vi "Get Default Configuration.vi"() -> (2 "Configuration":T1)   [LabVIEW 2014, in "System.lvclass"]
uses:
  System.lvclass
  Configuration - cluster.ctl
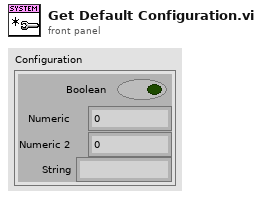
[diagram p1: front panel]
types:
  T1 = typedef "System.lvclass/Configuration - cluster.ctl" = cluster{"Boolean":bool, "Numeric":dbl, "Numeric 2":dbl, "String":string}
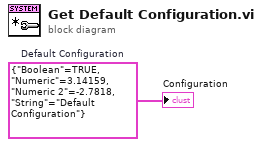
[diagram p0: block diagram]
diagram:
  w1 = T1 {"Boolean"=TRUE, "Numeric"=3.14159, "Numeric 2"=-2.7818, "String"="Default Configuration"}  # Default Configuration
  "Configuration" <- w1
